vi "ShowHelpPages.vi"() -> ()   [LabVIEW 2014]
panel:
  in  "Done":bool
  out "image":picture
  in  "Listbox":i32(listbox)
  # "How Do I?"
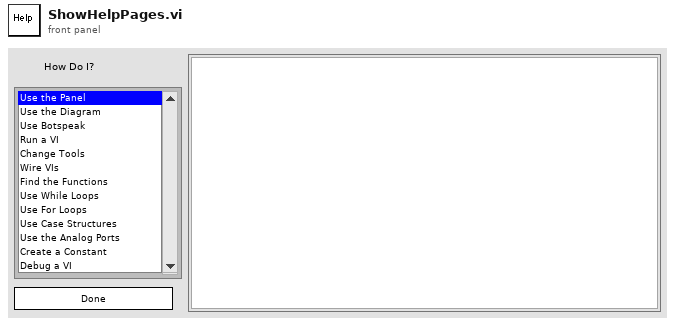
[diagram p1: front panel]
types:
  T1 = typedef "LVBoundsTypeDef.ctl" = cluster{"Width":u32, "Height":u32}
  T2 = typedef "QT_Image.ctl" = cluster{"Width":i32, "Height":i32, "Depth":i32, "data":u8[], "Compressed data":u8[], "Color table":u32[], "Duration":i32, "Options":i32, "Timestamp":i32, "ID":i32, "Reserved":i32, "Dialogs":u32}
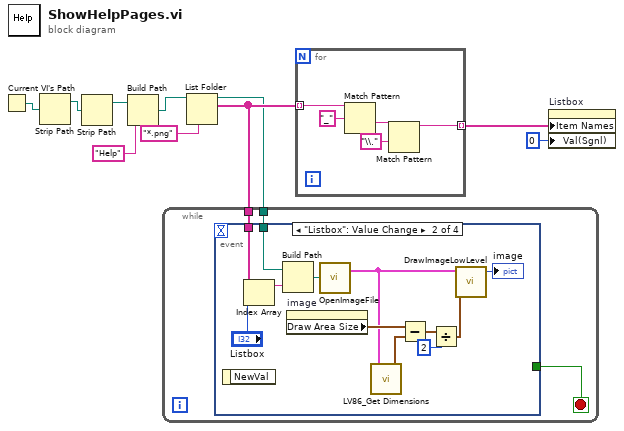
[diagram p0: block diagram]
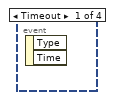
[diagram p2: hidden frame]
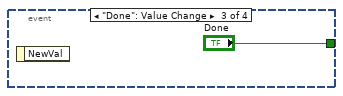
[diagram p3: hidden frame]
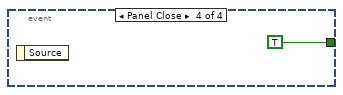
[diagram p4: hidden frame]
diagram:
  n1 = Current VI's Path() -> (path=w10:path)
  n2 = Strip Path(path=w10) -> (stripped path=w9:path)  [unwired: 1 out]
  n3 = Strip Path(path=w9) -> (stripped path=w8:path)  [unwired: 1 out]
  n4 = Build Path(base path=w8, name or relative path="Help") -> (appended path=w6:path)
  n5 = List Folder(path=w6, pattern="*.png") -> (path out=w2:path, filenames=w3:string[])  [unwired: 2 in, 2 out]
  n6 = while {
    tunnel: w3 -> [w13]
    tunnel: w2 -> [w12]
    stop <- w11 stop-if-true
    n7 = event shown="[1] \"Listbox\": Value Change" {
      selector: _ -> [_ _ _ _]
      dyn-events: _ -> [_ _ _ _]
      timeout: _ -> [_ _ _ _]
      tunnel: w13 -> [_ w24 _ _]
      tunnel: w12 -> [_ w22 _ _]
      tunnel: [_ _ "Done" TRUE ("Done")] -> w11
      event Timeout {
        n8 = event-data() -> ()  [unwired: 1 in, 2 out]
      }
      event "Listbox": Value Change {
        n9 = event-data() -> ()  [unwired: 1 in, 1 out]
        n10 = Index Array(array=w24, index="Listbox") -> (element=w23:string)
        n11 = Build Path(base path=w22, name or relative path=w23) -> (appended path=w21:path)
        n12 = property on="image" class="Pict"() -> ("Draw Area Size"=w20:T1)  [unwired: 2 in, 2 out]
        n13 = call <userlib>:"OpenImageFile.vi"("selected path"=w21) -> ("Image Out"=w16:T2)  [unwired: 2 in]
        n14 = call <userlib>:"LV86_Get Dimensions.vi"("Image In"=w16) -> ("Dimensions"=w19:cluster{"Width":i32, "Height":i32})  [unwired: 1 in, 1 out]
        n15 = Subtract(x=w20, y=w19) -> (x-y=w18:T1)
        n16 = Divide(x=w18, y=2) -> (x/y=w14:cluster{"Width":dbl, "Height":dbl})
        n17 = call <userlib>:"DrawImageLowLevel.vi"("Image"=w16, "Position"=w14) -> ("new picture"=→"image":picture)  [unwired: 3 in, 1 out]
      }
      event "Done": Value Change {
        n18 = event-data() -> ()  [unwired: 1 in, 1 out]
      }
      event Panel Close {
        n19 = event-data() -> ()  [unwired: 1 in, 1 out]
      }
    }
  }
  n20 = for {
    tunnel: w3 -> [w32] mode=indexing
    tunnel: [w28] -> w4 mode=indexing
    n21 = Match Pattern(string=w32, regular expression="_") -> (after substring=w30:string)  [unwired: 1 in, 3 out]
    n22 = Match Pattern(string=w30, regular expression="\\.") -> (before substring=w28:string)  [unwired: 1 in, 3 out]
  }
  n23 = property on="Listbox" class="LstBox (strict)"("Item Names"=w4, "Val(Sgnl)"=0 ("Value (Signaling)")) -> ()  [unwired: 2 in, 2 out]
